vi "test2.vi"() -> ()   [LabVIEW 2013]
uses:
  lightfield-automation-labview/VIs/ClientServerMode/CS_LFAClassGlobal.vi
  lightfield-automation-labview/LightField Automation.lvclass
panel:
  out "Intensity Graph":dbl[][](graph)
  out "x-y":dbl
  out "Waveform Graph":dbl[](graph)
  out "# elements in queue":i32
  in  "stop":bool
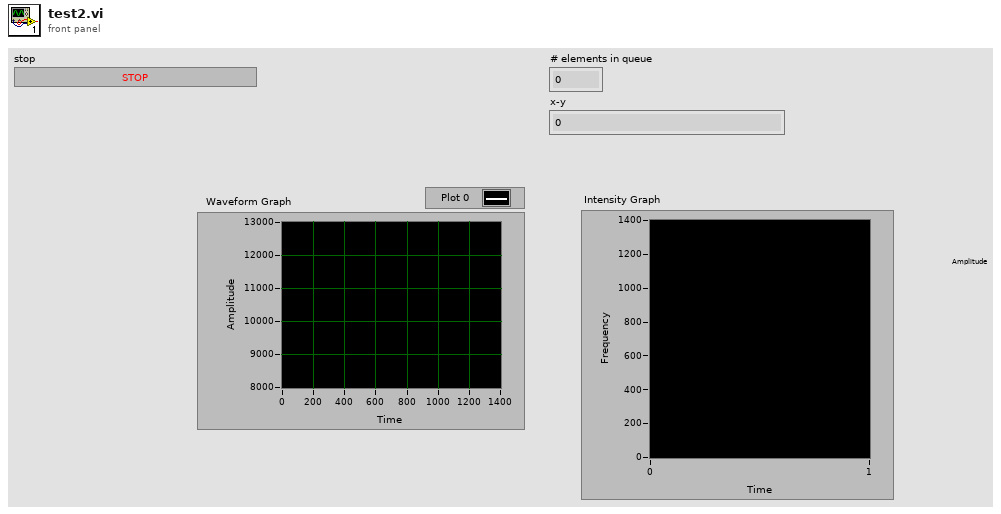
[diagram p1: front panel]
types:
  T1 = cluster{"Image":dbl[][][], "Frame Size":cluster{"F":i32, "Y":i32, "X":i32}}[]
  T2 = cluster{"Image":dbl[][][], "Frame Size":cluster{"F":i32, "Y":i32, "X":i32}}
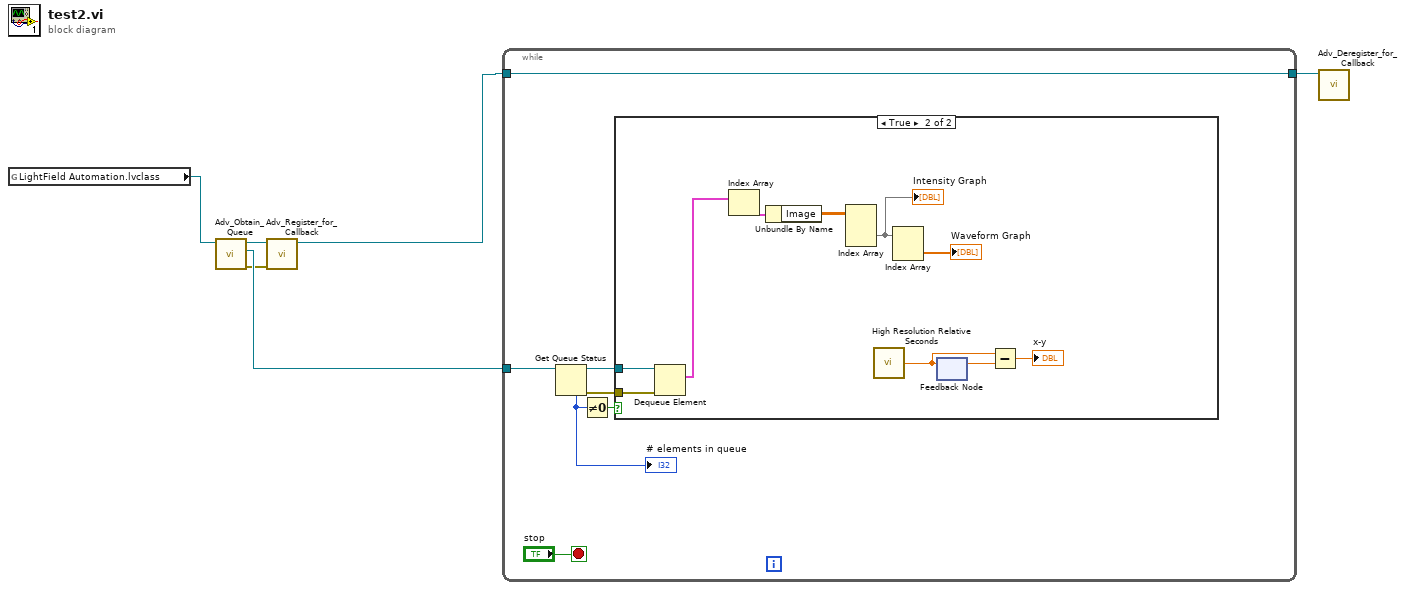
[diagram p0: block diagram]
diagram:
  n1 = global read "CS_LFAClassGlobal.vi" "LightField Automation.lvclass"() -> (w6:refnum<class "LightField Automation.lvclass">)
  n2 = call "Adv_Obtain_Queue.vi"("LightField Automation in"=w6) -> ("error out"=w3:errorcluster, "Queue Reference"=w4:refnum<queue>, "LightField Automation out"=w5:refnum<class "LightField Automation.lvclass">)  [unwired: 8 in]
  n3 = call "Adv_Register_for_Callback.vi"("error in (no error)"=w3, "LightField Automation in"=w5) -> ("LightField Automation out"=w2:refnum<class "LightField Automation.lvclass">)  [unwired: 8 in, 1 out]
  n4 = while {
    tunnel: w4 -> [w12]
    tunnel: w2 -> [w7]
    tunnel: [w7] -> w1
    stop <- "stop" stop-if-true
    n5 = Get Queue Status(queue=w12) -> (queue out=w11:refnum<queue>, error out=w10:errorcluster, # elements in queue=w8:i32)  [unwired: 2 in, 5 out]
    "# elements in queue" <- w8
    n6 = Not Equal To 0?(x=w8) -> (x != 0?=w9:bool)
    n7 = case shown="True" w9 {
      tunnel: w11 -> [_ w23]
      tunnel: w10 -> [_ w22]
      frame False {
      }
      frame True {
        n8 = Dequeue Element(queue=w23, error in (no error)=w22) -> (element=w21:T1)  [unwired: 1 in, 3 out]
        n9 = Index Array(array=w21) -> (element=w20:T2)  [unwired: 1 in]
        n10 = Unbundle By Name(w20) -> ("Image"=w19:dbl[][][])
        n11 = Index Array(array=w19) -> (element=w14:dbl[][])  [unwired: 3 in]
        "Intensity Graph" <- w14
        n12 = call <vilib>:"High Resolution Relative Seconds.vi"() -> ("relative seconds"=w16:dbl)
        n13 = Index Array(array=w14) -> (element=→"Waveform Graph":dbl[])  [unwired: 2 in]
        n14 = feedback-in #1(w16) -> ()
        n15 = feedback #1() -> (w17:dbl)  [unwired: 1 in]
        n16 = Subtract(x=w16, y=w17) -> (x-y=→"x-y":dbl)
      }
    }
  }
  n17 = call "Adv_Deregister_for_Callback.vi"("LightField Automation in"=w1) -> ()  [unwired: 9 in, 2 out]
